vi "Generate sorted scan parameters.vi"(2 "Scan parameters":T3(array[cluster])=[{"DAQ Channel"=2, "Label"="\nscaledVsg1=", "Scaled low"=-0.060000000000000005, "Scaled high"=0.14, "Start"=0.14, "End"=-0.060000000000000005, "Step"=-0.060000000000000005, "Scale?"=TRUE}, {"DAQ Channel"=2, "Label"="\nscaledVsg1=", "Scaled low"=-0.060000000000000005, "Scaled high"=0.14, "Start"=0.14, "End"=-0.060000000000000005, "Step"=-0.060000000000000005, "Scale?"=TRUE}, {"DAQ Channel"=2, "Label"="\nscaledVsg1=", "Scaled low"=-0.060000000000000005, "Scaled high"=0.14, "Start"=0.14, "End"=-0.060000000000000005, "Step"=-0.060000000000000005, "Scale?"=TRUE}, {"DAQ Channel"=3, "Label"="\nscaledVsg1=", "Scaled low"=-0.060000000000000005, "Scaled high"=0.14, "Start"=0.14, "End"=-0.060000000000000005, "Step"=-0.060000000000000005, "Scale?"=TRUE}] {"Step" format="%#_6p"; "End" format="%#_6p"; "Start" format="%#_6p"; "Scaled high" format="%#_6p"; "Scaled low" format="%#_6p"}, 3 "Scan control":cluster{"Priority":u16, "Scan name":u16}[](array[cluster])=[{"Priority"=1, "Scan name"=1}, {"Priority"=2, "Scan name"=2}, {"Priority"=0, "Scan name"=3}, {"Priority"=2, "Scan name"=4}] {"Scan name" items=["OFF", "Vsg1", "Vsg2", "Vsgw", "Vbg", "Field", "Temp"]; "Priority" items=["Priority 0", "Priority 1", "Priority 2", "Priority 3", "Priority 4", "Priority 5"]}) -> (0 "Sorted scan parameters":T1(array[cluster])=[{[{"DAQ Channel"=2, "Label"="\nscaledVsg1=", "Scaled low"=-0.060000000000000005, "Scaled high"=0.14, "Start"=0.14, "End"=-0.060000000000000005, "Step"=-0.060000000000000005, "Scale?"=TRUE}]}, {[{"DAQ Channel"=2, "Label"="\nscaledVsg1=", "Scaled low"=-0.060000000000000005, "Scaled high"=0.14, "Start"=0.14, "End"=-0.060000000000000005, "Step"=-0.060000000000000005, "Scale?"=TRUE}]}, {[{"DAQ Channel"=2, "Label"="\nscaledVsg1=", "Scaled low"=-0.060000000000000005, "Scaled high"=0.14, "Start"=0.14, "End"=-0.060000000000000005, "Step"=-0.060000000000000005, "Scale?"=TRUE}, {"DAQ Channel"=3, "Label"="\nscaledVsg1=", "Scaled low"=-0.060000000000000005, "Scaled high"=0.14, "Start"=0.14, "End"=-0.060000000000000005, "Step"=-0.060000000000000005, "Scale?"=TRUE}]}], 1 "Sorted scan control":T2(array[cluster])=[{[{"Priority"=0, "Scan name"=3}]}, {[{"Priority"=1, "Scan name"=1}]}, {[{"Priority"=2, "Scan name"=2}, {"Priority"=2, "Scan name"=4}]}])   [LabVIEW 2013]
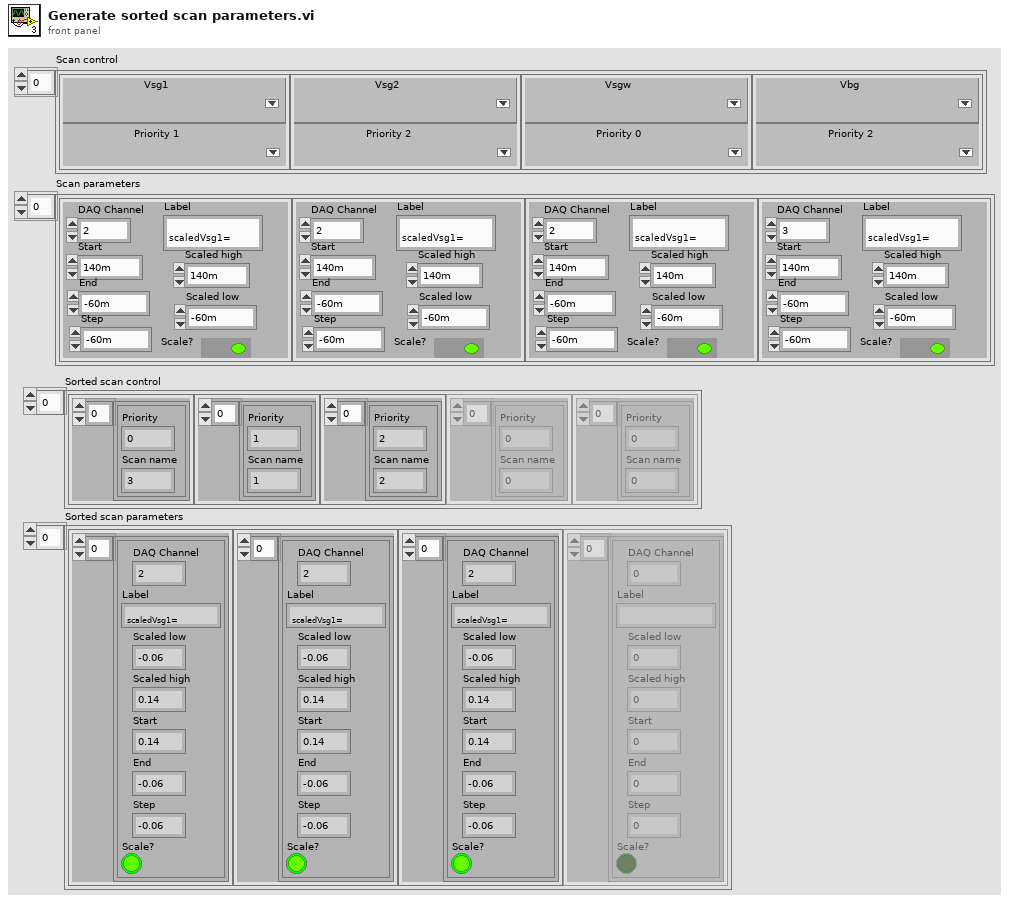
[diagram p1: front panel]
types:
  T1 = cluster{cluster{"DAQ Channel":i32, "Label":string, "Scaled low":dbl, "Scaled high":dbl, "Start":dbl, "End":dbl, "Step":dbl, "Scale?":bool}[]}[]
  T2 = cluster{cluster{"Priority":u16, "Scan name":u16}[]}[]
  T3 = cluster{"DAQ Channel":i32, "Label":string, "Scaled low":dbl, "Scaled high":dbl, "Start":dbl, "End":dbl, "Step":dbl, "Scale?":bool}[]
  T4 = cluster{"DAQ Channel":i32, "Label":string, "Scaled low":dbl, "Scaled high":dbl, "Start":dbl, "End":dbl, "Step":dbl, "Scale?":bool}
  T5 = cluster{cluster{"DAQ Channel":i32, "Label":string, "Scaled low":dbl, "Scaled high":dbl, "Start":dbl, "End":dbl, "Step":dbl, "Scale?":bool}[]}
  T6 = cluster{cluster{"Priority":u16, "Scan name":u16}[]}
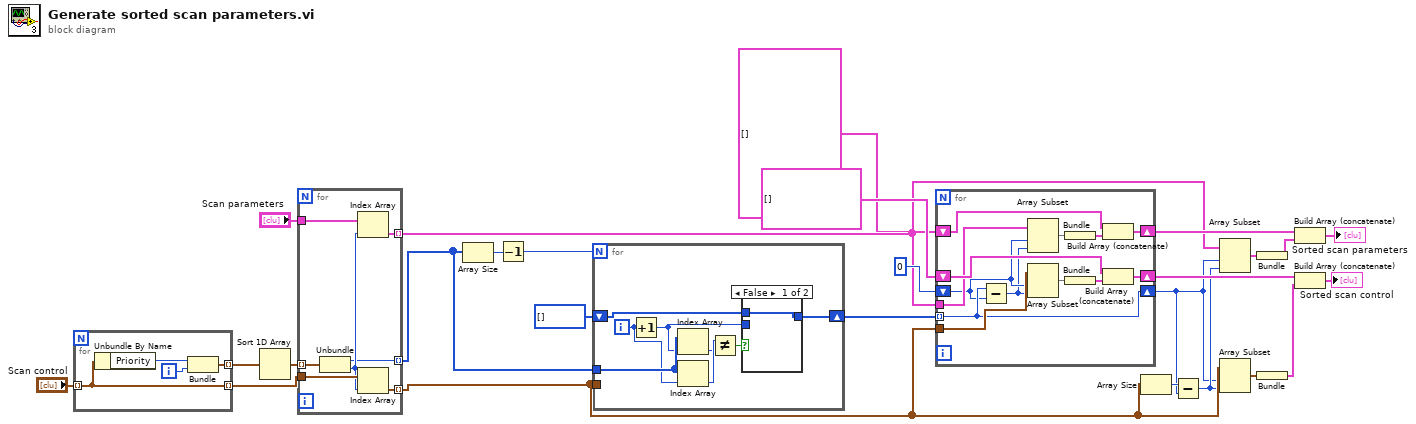
[diagram p0: block diagram]
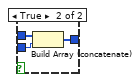
[diagram p2: hidden frame]
diagram:
  n1 = for {
    tunnel: "Scan control" -> [w27] mode=indexing
    tunnel: [w30] -> w25 mode=indexing
    tunnel: [w27] -> w23 mode=indexing
    i -> [w28]
    n2 = Unbundle By Name(w27) -> ("Priority"=w29:u16)
    n3 = Bundle("Priority"=w29, w28) -> (w30:cluster{"Priority":u16, i32})  [unwired: 1 in]
  }
  n4 = Sort 1D Array(array=w25) -> (sorted array=w24:cluster{"Priority":u16, i32}[])
  n5 = for {
    tunnel: w24 -> [w37] mode=indexing
    tunnel: w23 -> [w36]
    tunnel: [w35] -> w11 mode=indexing
    tunnel: "Scan parameters" -> [w34]
    tunnel: [w33] -> w6 mode=indexing
    tunnel: [w31] -> w19 mode=indexing
    n6 = Unbundle(w37) -> ("Priority"=w31:u16, w32:i32)
    n7 = Index Array(array=w34, index=w32) -> (element=w33:T4)
    n8 = Index Array(array=w36, index=w32) -> (element=w35:cluster{"Priority":u16, "Scan name":u16})
  }
  n9 = Array Size(array=w19) -> (size(s)=w21:i32)
  n10 = Decrement(x=w21) -> (x-1=w20:i32)
  n11 = for {
    N: w20 -> [_]
    tunnel: w19 -> [w45]
    shift-right: [w41] -> w16
    shift-left: u16[] [] -> [w40]
    tunnel: w11 -> [_]
    i -> [w38]
    n12 = Increment(x=w38) -> (x+1=w39:i32)
    n13 = Index Array(array=w45, index=w39) -> (element=w42:u16)
    n14 = Index Array(array=w45, index=w38) -> (element=w44:u16)
    n15 = Not Equal?(x=w44, y=w42) -> (x != y?=w43:bool)
    n16 = case shown="False" w43 {
      tunnel: [w46 w49] -> w41
      tunnel: w40 -> [w46 w48]
      tunnel: w39 -> [_ w47]
      frame False {
      }
      frame True {
        n17 = Build Array (concatenate)(w48, w47) -> (w49:i32[])
      }
    }
  }
  n18 = for {
    tunnel: w16 -> [w57] mode=indexing
    shift-right: [w62] -> w15
    shift-left: T2 [] -> [w61]
    tunnel: w11 -> [w60]
    shift-right: [w57] -> w4
    shift-left: 0 -> [w55]
    tunnel: w6 -> [w56]
    shift-right: [w52] -> w7
    shift-left: T1 [] -> [w51]
    n19 = Subtract(x=w57, y=w55) -> (x-y=w54:i32)
    n20 = Array Subset(array=w56, index=w55, length=w54) -> (w53:T3)
    n21 = Array Subset(array=w60, index=w55, length=w54) -> (w59:cluster{"Priority":u16, "Scan name":u16}[])
    n22 = Bundle(w53) -> (w50:T5)  [unwired: 1 in]
    n23 = Bundle(w59) -> (w58:T6)  [unwired: 1 in]
    n24 = Build Array (concatenate)(w51, w50) -> (w52:T1)
    n25 = Build Array (concatenate)(w61, w58) -> (w62:T2)
  }
  n26 = Array Size(array=w11) -> (size(s)=w12:i32)
  n27 = Subtract(x=w12, y=w4) -> (x-y=w5:i32)
  n28 = Array Subset(array=w6, index=w4, length=w5) -> (w8:T3)
  n29 = Array Subset(array=w11, index=w4, length=w5) -> (w10:cluster{"Priority":u16, "Scan name":u16}[])
  n30 = Bundle(w8) -> (w2:T5)  [unwired: 1 in]
  n31 = Bundle(w10) -> (w9:T6)  [unwired: 1 in]
  n32 = Build Array (concatenate)(w7, w2) -> (→"Sorted scan parameters":T1)
  n33 = Build Array (concatenate)(w15, w9) -> (→"Sorted scan control":T2)
